vi "LCC Set PID Parameter.vi"(7 "PID Parameter ID":T1 items=["PID_PARAM_K", "PID_PARAM_T_I", "PID_PARAM_T_D", "PID_PARAM_DERIVATIVE_GAIN_LIMIT", "PID_PARAM_T_T", "PID_PARAM_MAX_U", "PID_PARAM_MIN_U", "PID_PARAM_DISABLED_U", "PID_PARAM_INITIAL_SETPOINT", "PID_PARAM_SAMPLE_TIME"], 8 "error in (no error)":errorcluster caption="Fehler (Eingang, kein Fehler)", 10 "Value":dbl, 11 "ChanHdl":i64) -> (0 "error out":errorcluster caption="Fehler (Ausgang)")   [LabVIEW 2021, in "labbCAN_Controller_API.lvlib"]
doc: "LCC_Func long LCC_CALL LCC_SetPIDParameter(dev_hdl ChanHdl, int PIDParamId,\n double Value);"
uses:
  labbCAN_Controller_API.lvlib
  PIDParameterId.ctl
  labbCAN_Controller_API.dll
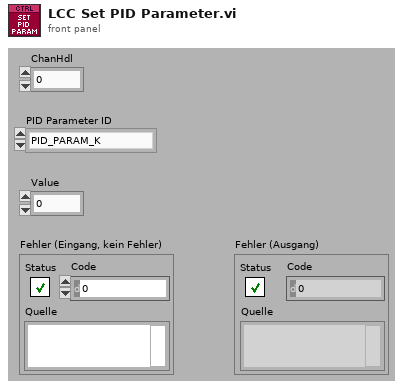
[diagram p1: front panel]
types:
  T1 = typedef "labbCAN_Controller_API.lvlib/PIDParameterId.ctl" = i32
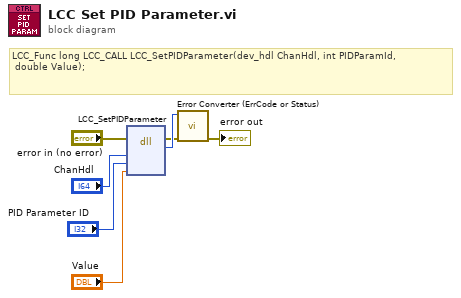
[diagram p0: block diagram]
diagram:
  # "LCC_Func long LCC_CALL LCC_SetPIDParameter(dev_hdl ChanHdl, int PIDParamId,\n\tdouble Value);"
  n1 = dll-call lib="C:/Users/olaja/AppData/Local/CETONI_SDK/labbCAN_Controller_API.*" fn="LCC_SetPIDParameter"(error in="error in (no error)", "ChanHdl"="ChanHdl", "PIDParamId"="PID Parameter ID", "Value"="Value") -> (error out=w3:errorcluster, "Rückgabetyp"=w4:i32)  [unwired: 5 in, 1 out]
  n2 = call "Error Converter (ErrCode or Status).vi"("error in (no error)"=w3, "error code"=w4) -> ("error out"=→"error out":errorcluster)  [unwired: 9 in]
